vi "运维调试_五参数.vi"(11 "编号":string) -> ()   [LabVIEW 2016, in "斯坦道多参数.lvlib"]
uses:
  <vilib>/Utility/miscctls.llb/LVPointTypeDef.ctl
  <vilib>/Plasmionique/MB Master/MB_Master/MB_Master.lvclass
  <vilib>/Utility/config.llb/NI_LVConfig.lvlib
  <vilib>/ptbypt/NI_PtbyPt.lvlib
panel:
  in  "探头设置":bool
  in  "量程设置":bool
  out "簇":T1
  in  "传感器系列号":bool
  in  "水样保存组数":dbl caption="水样保存组数:"
  in  "水样稳定时间":dbl caption="水样稳定时间:"
  out "模块版本号":string
  out "权限等级":string
  in  "打开modbus":bool
  out "选项卡控件":enum32{"选项卡 1", "选项卡 2"}(tab)
  in  "VISA资源名称":refnum<visa-resource-name> caption="串口"
  in  "IP":string="localhost" caption="IP:"
  in  "Port":u16=502 caption="Port:"
  in  "自动断线重连":bool=TRUE
  in  "连接方式":u16(ring) items=["Modbus RTU", "Modbus TCP"]
  in  "密码锁":bool
  in  "设置页返回":bool
  in  "周期设置":bool
  out "当前串口":string
  out "运行状态":enum16{"空闲", "水样测试", "标样核查"}(ring)
  in  "停止":bool
  in  "标样核查":bool
  in  "水样测试":bool
  in  "设置":bool
  in  "探头校正返回":bool
  in  "探头校正":bool
  # "请设置仪器连接方式"
  # "组"
  # "min"
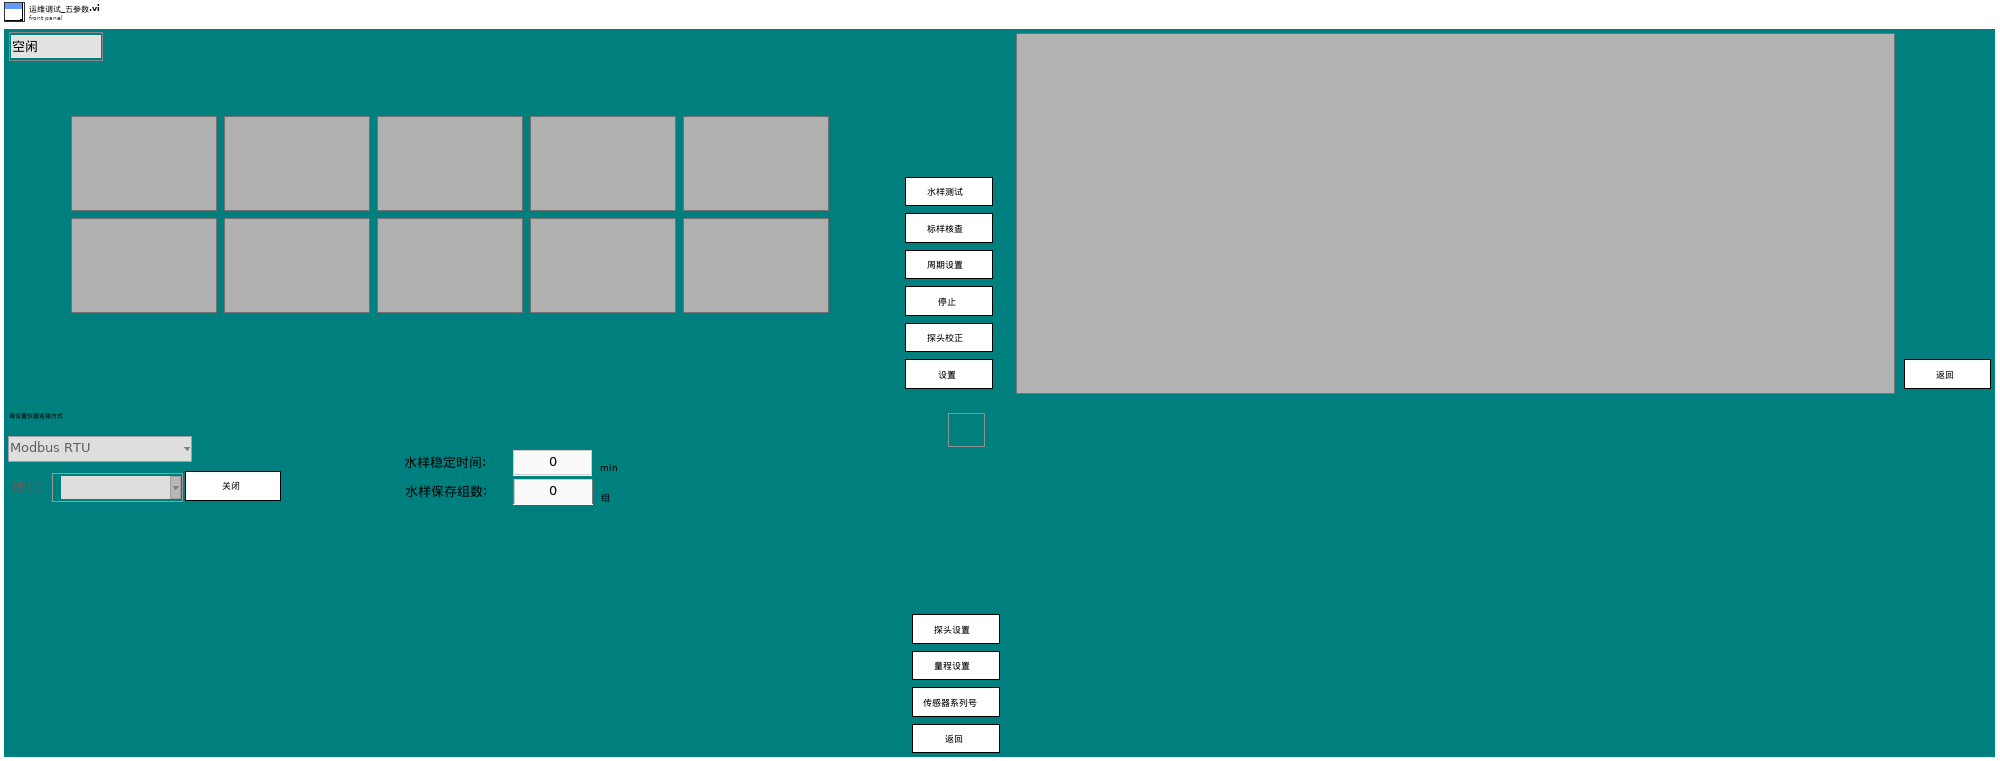
[diagram p1: front panel]
types:
  T1 = typedef "多状态显示框.ctl" = cluster{"多参数状态显示":cluster{"标签":string, "检测值1":cluster{"检测值":dbl, "单位":string, "启用":bool}, "检测值2":cluster{"检测值":dbl, "单位":string, "启用":bool}, "数据标识":string}, "多参数状态显示 2":cluster{"标签":string, "检测值1":cluster{"检测值":dbl, "单位":string, "启用":bool}, "检测值2":cluster{"检测值":dbl, "单位":string, "启用":bool}, "数据标识":string}, "多参数状态显示 3":cluster{"标签":string, "检测值1":cluster{"检测值":dbl, "单位":string, "启用":bool}, "检测值2":cluster{"检测值":dbl, "单位":string, "启用":bool}, "数据标识":string}, "多参数状态显示 4":cluster{"标签":string, "检测值1":cluster{"检测值":dbl, "单位":string, "启用":bool}, "检测值2":cluster{"检测值":dbl, "单位":string, "启用":bool}, "数据标识":string}, "多参数状态显示 5":cluster{"标签":string, "检测值1":cluster{"检测值":dbl, "单位":string, "启用":bool}, "检测值2":cluster{"检测值":dbl, "单位":string, "启用":bool}, "数据标识":string}, "多参数状态显示 6":cluster{"标签":string, "检测值1":cluster{"检测值":dbl, "单位":string, "启用":bool}, "检测值2":cluster{"检测值":dbl, "单位":string, "启用":bool}, "数据标识":string}, "多参数状态显示 7":cluster{"标签":string, "检测值1":cluster{"检测值":dbl, "单位":string, "启用":bool}, "检测值2":cluster{"检测值":dbl, "单位":string, "启用":bool}, "数据标识":string}, "多参数状态显示 8":cluster{"标签":string, "检测值1":cluster{"检测值":dbl, "单位":string, "启用":bool}, "检测值2":cluster{"检测值":dbl, "单位":string, "启用":bool}, "数据标识":string}, "多参数状态显示 9":cluster{"标签":string, "检测值1":cluster{"检测值":dbl, "单位":string, "启用":bool}, "检测值2":cluster{"检测值":dbl, "单位":string, "启用":bool}, "数据标识":string}, "多参数状态显示 10":cluster{"标签":string, "检测值1":cluster{"检测值":dbl, "单位":string, "启用":bool}, "检测值2":cluster{"检测值":dbl, "单位":string, "启用":bool}, "数据标识":string}}
  T2 = typedef "斯坦道多参数.lvlib/数据流类型.ctl" = cluster{"cmd":enum16{"水样测试", "标样核查", "校准状态同步", "停止"}, "data":variant}
  T3 = typedef "LVPointTypeDef.ctl" = cluster{"Horizontal":i16, "Vertical":i16}
  T4 = enum8{"Enabled", "Disabled", "Disabled and Grayed Out"}
  T5 = cluster{"标签":string, "检测值1":cluster{"检测值":dbl, "单位":string, "启用":bool}, "检测值2":cluster{"检测值":dbl, "单位":string, "启用":bool}, "数据标识":string}[]
  T6 = cluster{"标签":string, "检测值1":cluster{"检测值":dbl, "单位":string, "启用":bool}, "检测值2":cluster{"检测值":dbl, "单位":string, "启用":bool}, "数据标识":string}
  T7 = cluster{"CH":u16, "监测值":dbl, "信号值":sgl, "数据标识":string}
  T8 = cluster{"温度测量值":sgl, "测量值":sgl, "温度偏移修正值":sgl, "信号值":sgl, "数据标识":string}
  T9 = cluster{"温度测量值":sgl, "DO%":sgl, "DOmg/L":sgl, "温度偏移修正值":sgl, "数据标识mg/L":string, "数据标识%":string}
  T10 = cluster{"数组[0]":cluster{"标签":string, "检测值1":cluster{"检测值":dbl, "单位":string, "启用":bool}, "检测值2":cluster{"检测值":dbl, "单位":string, "启用":bool}, "数据标识":string}, "数组[1]":cluster{"标签":string, "检测值1":cluster{"检测值":dbl, "单位":string, "启用":bool}, "检测值2":cluster{"检测值":dbl, "单位":string, "启用":bool}, "数据标识":string}, "数组[2]":cluster{"标签":string, "检测值1":cluster{"检测值":dbl, "单位":string, "启用":bool}, "检测值2":cluster{"检测值":dbl, "单位":string, "启用":bool}, "数据标识":string}, "数组[3]":cluster{"标签":string, "检测值1":cluster{"检测值":dbl, "单位":string, "启用":bool}, "检测值2":cluster{"检测值":dbl, "单位":string, "启用":bool}, "数据标识":string}, "数组[4]":cluster{"标签":string, "检测值1":cluster{"检测值":dbl, "单位":string, "启用":bool}, "检测值2":cluster{"检测值":dbl, "单位":string, "启用":bool}, "数据标识":string}, "数组[5]":cluster{"标签":string, "检测值1":cluster{"检测值":dbl, "单位":string, "启用":bool}, "检测值2":cluster{"检测值":dbl, "单位":string, "启用":bool}, "数据标识":string}, "数组[6]":cluster{"标签":string, "检测值1":cluster{"检测值":dbl, "单位":string, "启用":bool}, "检测值2":cluster{"检测值":dbl, "单位":string, "启用":bool}, "数据标识":string}, "数组[7]":cluster{"标签":string, "检测值1":cluster{"检测值":dbl, "单位":string, "启用":bool}, "检测值2":cluster{"检测值":dbl, "单位":string, "启用":bool}, "数据标识":string}, "数组[8]":cluster{"标签":string, "检测值1":cluster{"检测值":dbl, "单位":string, "启用":bool}, "检测值2":cluster{"检测值":dbl, "单位":string, "启用":bool}, "数据标识":string}, "数组[9]":cluster{"标签":string, "检测值1":cluster{"检测值":dbl, "单位":string, "启用":bool}, "检测值2":cluster{"检测值":dbl, "单位":string, "启用":bool}, "数据标识":string}}
  T11 = cluster{"周期设置类型":enum16{"定点启动", "间隔启动"}, "定时功能启用":bool, "定时间隔":u32, "24H周期设置":bool[]}
  T12 = typedef "LVDateTimeRec.ctl" = cluster{"秒数的小数部分":dbl, "秒":i32, "分":i32, "时":i32, "日":i32, "月":i32, "年":i32, "天数（周）":i32, "天数（年）":i32, "DST":i32}
  T13 = cluster{"运行模式":enum16{"维护模式", "常规模式", "应急模式", "质控模式"}, "24H周期设置":bool[]}
  T14 = cluster{"Major":u16, "Minor":u16, "Fix":u16, "Build":u16}
  T15 = typedef "NI_LVConfig.lvlib/Config Data RefNum.ctl" = refnum<k1>
  T16 = enum32{"Bad", "Idle", "Run top level", "Running"}
  T17 = cluster{"ph":bool, "DO":bool, "Cond":bool, "Turb":bool, "叶绿素a":bool, "藻密度":bool, "ORP":bool, "cod":bool, "DO2":bool}
  T18 = cluster{"baud rate (bps)":u32, "stop bits":u16, "parity":u16, "flow control":u16, "timeout":u32, "retries":i32}
  T19 = cluster{"水温 (℃)":cluster{"量程下限":dbl, "量程上限":dbl}, "DO (mg/L)":cluster{"量程下限":dbl, "量程上限":dbl}, "DO (%)":cluster{"量程下限":dbl, "量程上限":dbl}, "pH":cluster{"量程下限":dbl, "量程上限":dbl}, "电导率 (μS/cm)":cluster{"量程下限":dbl, "量程上限":dbl}, "盐度":cluster{"量程下限":dbl, "量程上限":dbl}, "浊度 (NTU)":cluster{"量程下限":dbl, "量程上限":dbl}, "叶绿素a (μg/L)":cluster{"量程下限":dbl, "量程上限":dbl}, "藻密度 (cells/mL)":cluster{"量程下限":dbl, "量程上限":dbl}, "ORP (mV)":cluster{"量程下限":dbl, "量程上限":dbl}}
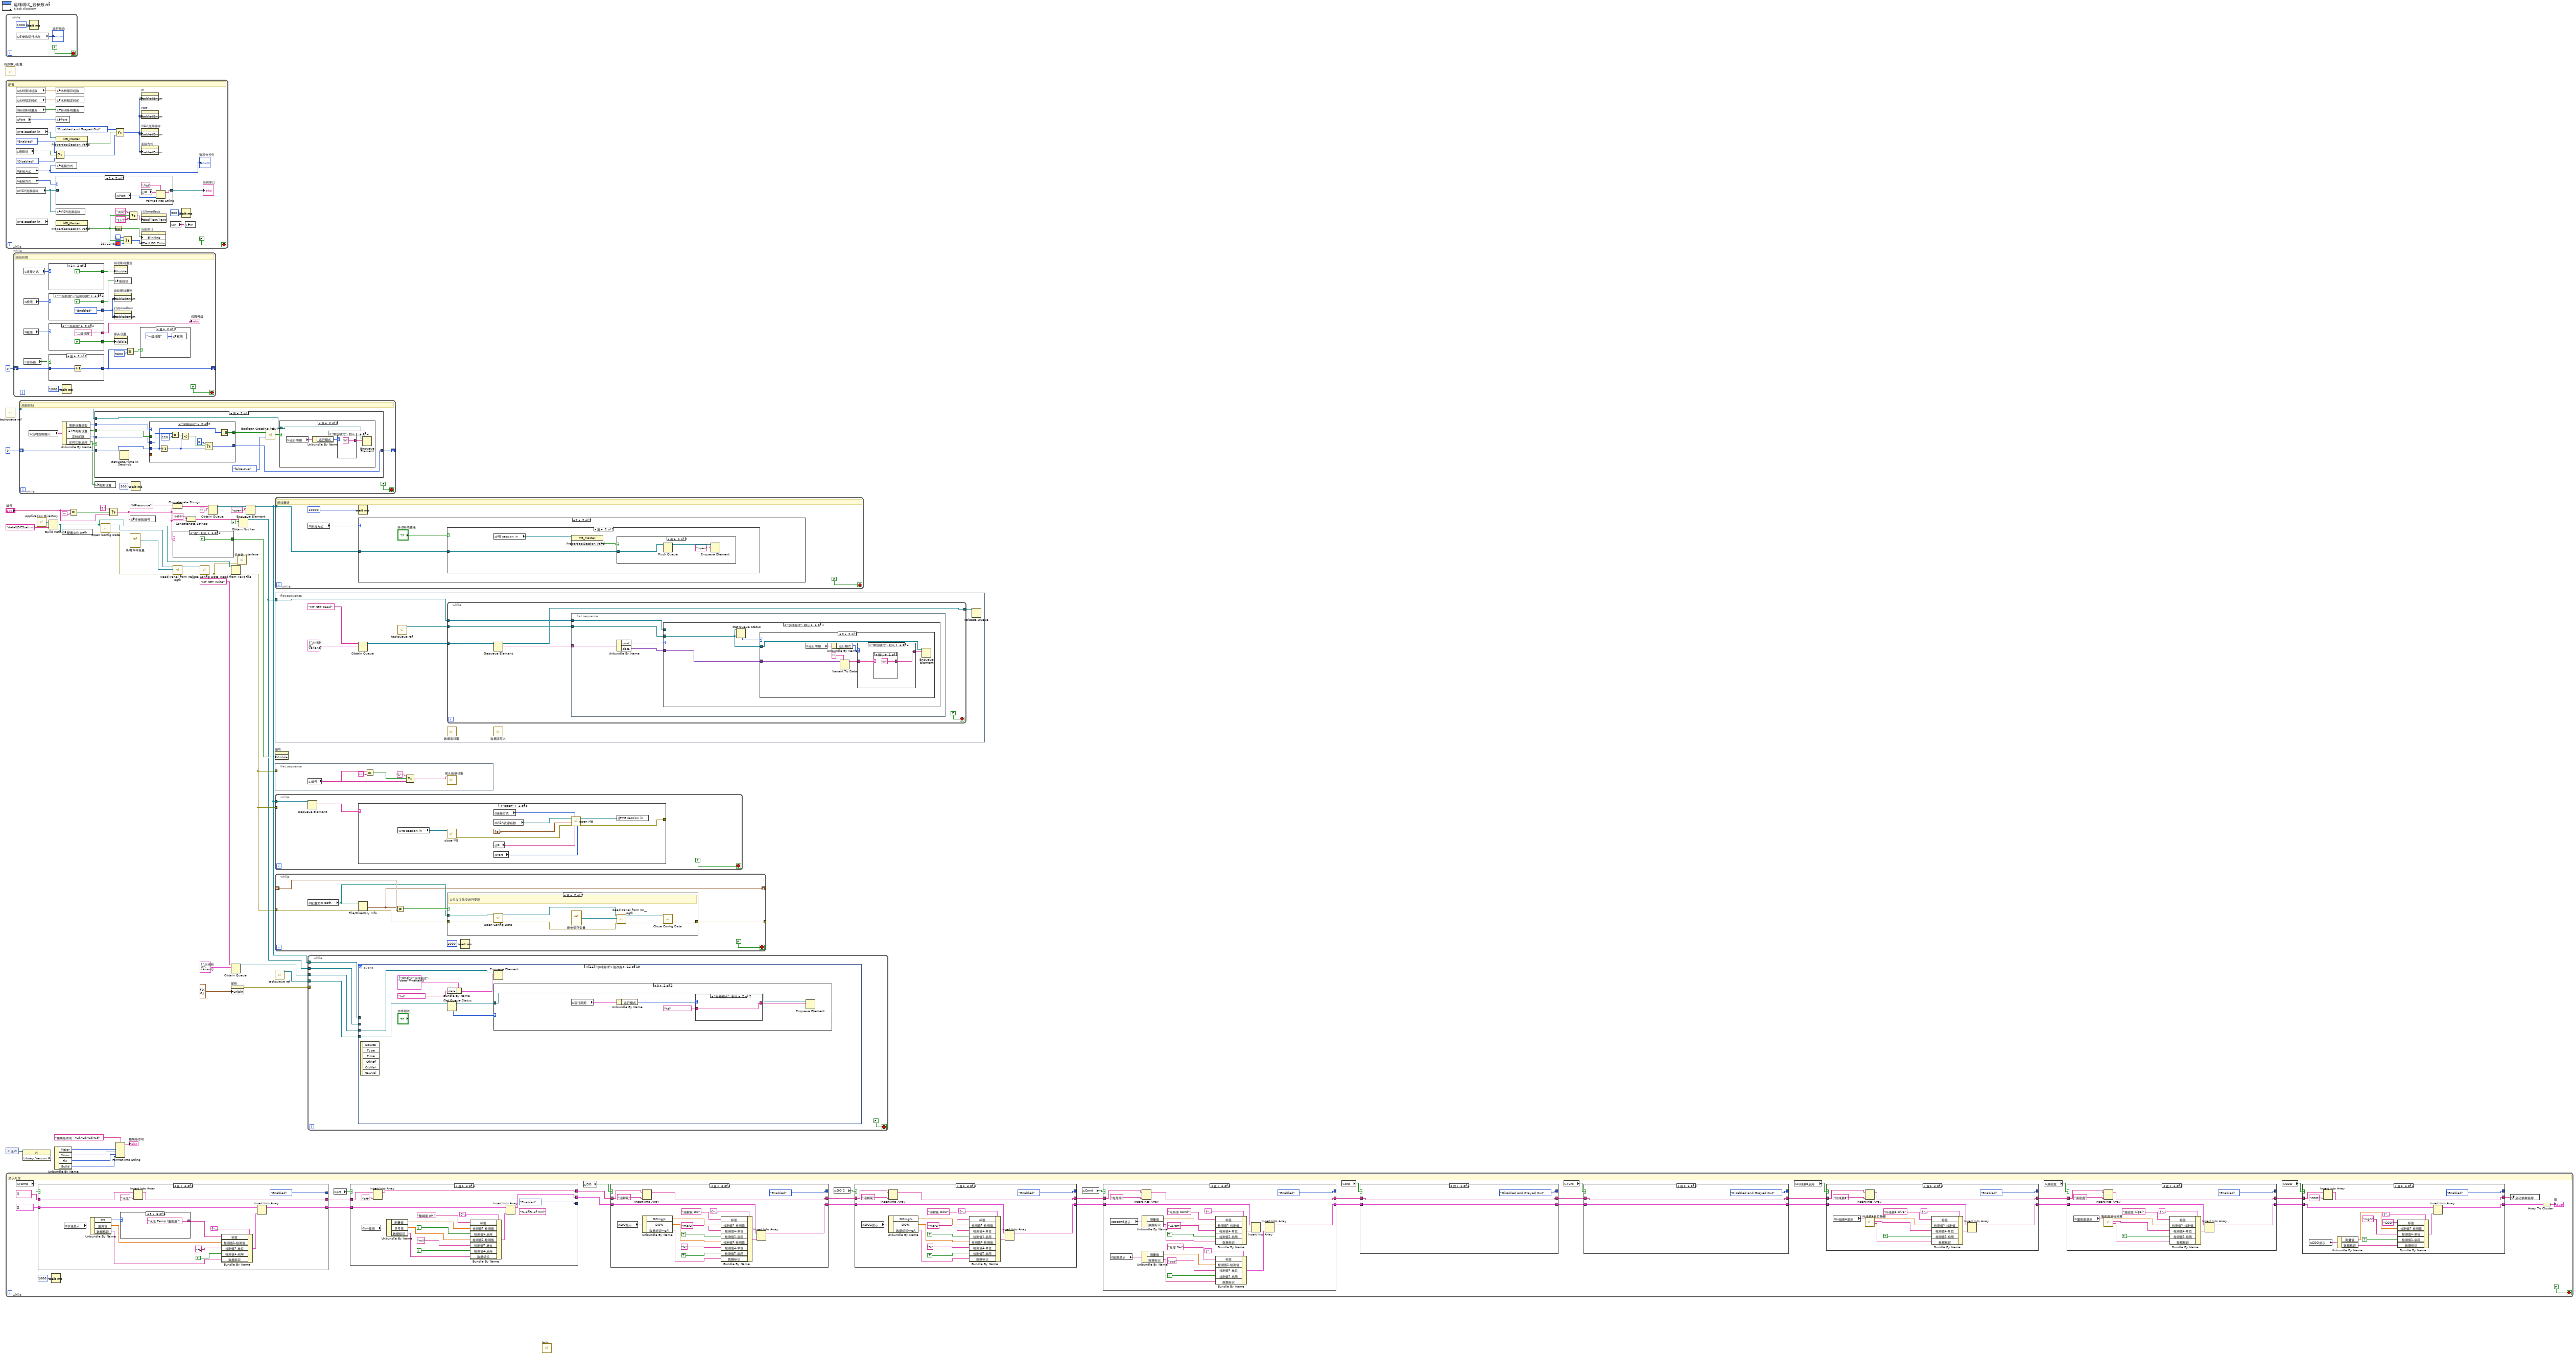
[diagram p0: block diagram]
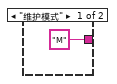
[diagram p3: hidden frame]
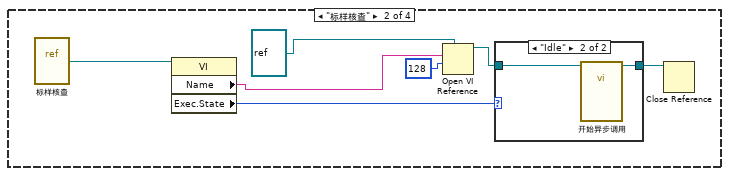
[diagram p5: hidden frame]
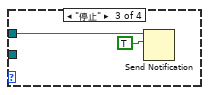
[diagram p7: hidden frame]
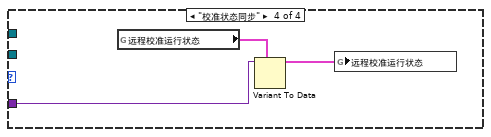
[diagram p8: hidden frame]
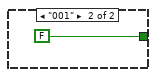
[diagram p9: hidden frame]
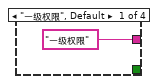
[diagram p17: hidden frame]
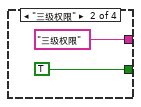
[diagram p18: hidden frame]
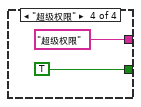
[diagram p19: hidden frame]
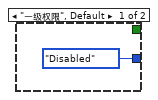
[diagram p20: hidden frame]
diagram:
  n1 = while {
    stop <- FALSE stop-if-true
    n2 = global read "多参数全局变量.vi" "多参数运行状态"() -> (→"运行状态":u16)
    n3 = Wait (ms)(milliseconds to wait=u32 1000 ("等待时间（毫秒）")) -> ()  [unwired: 1 out]
  }
  n4 = call "程序默认配置.vi"() -> ()  [unwired: 11 in, 1 out]
  n5 = while {
    stop <- FALSE stop-if-true
    # "配置"
    n6 = global read "断电保存变量.vi" "水样测试组数"() -> (w47:dbl)
    n7 = global read "断电保存变量.vi" "水样稳定时间"() -> (w49:dbl)
    n8 = global read "断电保存变量.vi" "自动断线重连"() -> (w50:bool)
    n9 = global read "断电保存变量.vi" "Port"() -> (w61:u16)
    n10 = global read "多参数全局变量.vi" "MB session in"() -> (w73:refnum<class "MB_Master.lvclass">)
    n11 = local read "密码锁"() -> (w66:bool)
    n12 = global read "断电保存变量.vi" "连接方式"() -> (w55:u16)
    "选项卡控件" <- w55
    n13 = global read "断电保存变量.vi" "连接方式"() -> (w59:u16)
    n14 = global read "断电保存变量.vi" "VISA资源名称"() -> (w58:refnum<visa-resource-name>)
    n15 = global read "多参数全局变量.vi" "MB session in"() -> (w70:refnum<class "MB_Master.lvclass">)
    n16 = Select(t=T4."Enabled" ("f"), s=w66, f=T4."Disabled") -> (s? t:f=w64:T4)
    n17 = local write "水样保存组数"(w47) -> ()
    n18 = local write "水样稳定时间"(w49) -> ()
    n19 = local write "自动断线重连"(w50) -> ()
    n20 = local write "Port"(w61) -> ()
    n21 = property class="MB_Master"(reference=w73) -> ("Properties:Session Valid"=w72:bool)  [unwired: 1 in, 2 out]
    n22 = local write "连接方式"(w55) -> ()
    n23 = case shown="1" w59 {
      tunnel: w58 -> [w75 _]
      tunnel: [w75 w76] -> w57
      frame 0, Default {
      }
      frame 1 {
        n24 = global read "断电保存变量.vi" "Port"() -> (w77:u16)
        n25 = global read "断电保存变量.vi" "IP"() -> (w79:string)
        n26 = Format Into String(format string=":%d" ("格式字符串"), initial string=w79, w77) -> (resulting string=w76:string)  [unwired: 1 in, 1 out]
      }
    }
    "当前串口" <- w57
    n27 = local write "VISA资源名称"(w58) -> ()
    n28 = property class="MB_Master"(reference=w70) -> ("Properties:Session Valid"=w54:bool)  [unwired: 1 in, 2 out]
    n29 = Not(x=w54) -> (.not. x?=w56:bool)
    n30 = Select(t=T4."Disabled and Grayed Out" ("禁用"), s=w72, f=w64) -> (s? t:f=w60:T4)
    n31 = Select(t=u32 16777216, s=w54, f=u32 16722483) -> (s? t:f=w51:u32)
    n32 = Select(t="关闭" ("布尔文本.文本"), s=w54, f="打开" ("布尔文本.文本")) -> (s? t:f=w67:string)
    n33 = property on="IP" class="Str"("DisabledEnum"=w60) -> ()  [unwired: 2 in, 2 out]
    n34 = property on="Port" class="DigNum (严格)"("DisabledEnum"=w60) -> ()  [unwired: 2 in, 2 out]
    n35 = property on="VISA资源名称" class="VISAName"("DisabledEnum"=w60) -> ()  [unwired: 2 in, 2 out]
    n36 = property on="连接方式" class="Ring (严格)"("DisabledEnum"=w60) -> ()  [unwired: 2 in, 2 out]
    n37 = property on="打开modbus" class="Bool"("BoolText.Text"=w67) -> ()  [unwired: 2 in, 2 out]
    n38 = property on="当前串口" class="Str"("Blinking"=w56, "Text.BG Color"=w51) -> ()  [unwired: 2 in, 2 out]
    n39 = global read "断电保存变量.vi" "IP"() -> (w62:string)
    n40 = Wait (ms)(milliseconds to wait=u32 500 ("等待时间（毫秒）")) -> ()  [unwired: 1 out]
    n41 = local write "IP"(w62) -> ()
  }
  n42 = call "taskqueue ref.vi"() -> ("队列输出"=w4:refnum<queue>)  [unwired: 10 in, 1 out]
  n43 = control-ref of="本VI"() -> (w23:refnum<vi>)
  n44 = while {
    stop <- FALSE stop-if-true
    # "显示处理"
    n45 = global read "断电保存变量.vi" "Temp"() -> (w112:bool)
    n46 = case shown="真" w112 {
      tunnel: [w287 w299] -> w109
      tunnel: T5 [] ("数组") -> [w287 w300]
      tunnel: [T4."Disabled and Grayed Out" ("禁用") T4."Enabled" ("禁用")] -> _
      tunnel: string[] [] -> [w285 w290]
      tunnel: [w285 w289] -> w92
      frame False {
      }
      frame True {
        n47 = global read "多参数全局变量.vi" "水温显示"() -> (w297:T7)
        n48 = Unbundle By Name(w297) -> ("CH"=w296:u16, "监测值"=w294:dbl, "数据标识"=w293:string)
        n49 = case shown="5" w296 {
          tunnel: ["水温 Temp (pH)" ("监测参数1") "水温 Temp (DO)" ("监测参数1") "水温 Temp (浊度)" ("监测参数1") "水温 Temp (电导率)" ("监测参数1") "水温 Temp (叶绿素a)" ("监测参数1") "水温 Temp (藻密度)" ("监测参数1")] -> w302
          frame 0, Default {
          }
          frame 1 {
          }
          frame 2 {
          }
          frame 3 {
          }
          frame 4 {
          }
          frame 5 {
          }
        }
        n50 = Insert Into Array(array=w290, new element="水温" ("新元素/子数组")) -> (w289:string[])  [unwired: 1 in]
        n51 = Bundle By Name(cluster=T6 {"标签"="", "检测值1"={"检测值"=0.0, "单位"="", "启用"=FALSE}, "检测值2"={"检测值"=0.0, "单位"="", "启用"=FALSE}, "数据标识"=""} ("多参数状态显示"), "标签"=w302, "检测值1.检测值"=w294, "检测值1.单位"="℃", "检测值1.启用"=TRUE, "数据标识"=w293) -> (w301:T6)
        n52 = Insert Into Array(array=w300, new element=w301) -> (w299:T5)  [unwired: 1 in]
      }
    }
    n53 = Wait (ms)(milliseconds to wait=u32 1000 ("等待时间（毫秒）")) -> ()  [unwired: 1 out]
    n54 = global read "断电保存变量.vi" "pH"() -> (w110:bool)
    n55 = case shown="真" w110 {
      tunnel: [w268 w283] -> w107
      tunnel: w109 -> [w268 w284]
      tunnel: [T4."Disabled and Grayed Out" ("禁用") T4."Enabled" ("禁用")] -> _
      tunnel: w92 -> [w266 w271]
      tunnel: [w266 w270] -> w91
      frame False {
      }
      frame True {
        (unwired) "%.2f(%.2f mV)" ("格式字符串")
        n56 = global read "多参数全局变量.vi" "ph显示"() -> (w281:T8)
        n57 = Insert Into Array(array=w271, new element="pH" ("新元素/子数组")) -> (w270:string[])  [unwired: 1 in]
        n58 = Unbundle By Name(w281) -> ("测量值"=w278:sgl, "信号值"=w276:sgl, "数据标识"=w274:string)
        n59 = Bundle By Name(cluster=T6 {"标签"="", "检测值1"={"检测值"=0.0, "单位"="", "启用"=FALSE}, "检测值2"={"检测值"=0.0, "单位"="", "启用"=FALSE}, "数据标识"=""} ("多参数状态显示"), "标签"="酸碱度 pH" ("监测参数2"), "检测值1.检测值"=w278, "检测值1.启用"=TRUE, "检测值2.检测值"=w276, "检测值2.单位"="mV", "检测值2.启用"=TRUE, "数据标识"=w274) -> (w272:T6)
        n60 = Insert Into Array(array=w284, new element=w272) -> (w283:T5)  [unwired: 1 in]
      }
    }
    n61 = global read "断电保存变量.vi" "DO"() -> (w108:bool)
    n62 = case shown="真" w108 {
      tunnel: [w248 w264] -> w83
      tunnel: w107 -> [w248 w265]
      tunnel: [T4."Disabled and Grayed Out" ("禁用") T4."Enabled" ("禁用")] -> _
      tunnel: w91 -> [w246 w251]
      tunnel: [w246 w250] -> w82
      frame False {
      }
      frame True {
        n63 = global read "多参数全局变量.vi" "DO显示"() -> (w262:T9)
        n64 = Insert Into Array(array=w251, new element="溶解氧" ("新元素/子数组")) -> (w250:string[])  [unwired: 1 in]
        n65 = Unbundle By Name(w262) -> ("DOmg/L"=w259:sgl, "DO%"=w257:sgl, "数据标识mg/L"=w256:string)
        n66 = Bundle By Name(cluster=T6 {"标签"="", "检测值1"={"检测值"=0.0, "单位"="", "启用"=FALSE}, "检测值2"={"检测值"=0.0, "单位"="", "启用"=FALSE}, "数据标识"=""} ("多参数状态显示"), "标签"="溶解氧 DO" ("监测参数2"), "检测值1.检测值"=w259, "检测值1.单位"="mg/L", "检测值1.启用"=TRUE, "检测值2.检测值"=w257, "检测值2.单位"="%", "检测值2.启用"=TRUE, "数据标识"=w256) -> (w252:T6)
        n67 = Insert Into Array(array=w265, new element=w252) -> (w264:T5)  [unwired: 1 in]
      }
    }
    n68 = global read "断电保存变量.vi" "DO 2"() -> (w84:bool)
    n69 = case shown="真" w84 {
      tunnel: [w117 w133] -> w81
      tunnel: w83 -> [w117 w134]
      tunnel: [T4."Disabled and Grayed Out" ("禁用") T4."Enabled" ("禁用")] -> _
      tunnel: w82 -> [w115 w120]
      tunnel: [w115 w119] -> w80
      frame False {
      }
      frame True {
        n70 = global read "多参数全局变量.vi" "DO2显示"() -> (w131:T9)
        n71 = Insert Into Array(array=w120, new element="溶解氧" ("新元素/子数组")) -> (w119:string[])  [unwired: 1 in]
        n72 = Unbundle By Name(w131) -> ("DOmg/L"=w128:sgl, "DO%"=w126:sgl, "数据标识mg/L"=w125:string)
        n73 = Bundle By Name(cluster=T6 {"标签"="", "检测值1"={"检测值"=0.0, "单位"="", "启用"=FALSE}, "检测值2"={"检测值"=0.0, "单位"="", "启用"=FALSE}, "数据标识"=""} ("多参数状态显示"), "标签"="溶解氧 DO2" ("监测参数2"), "检测值1.检测值"=w128, "检测值1.单位"="mg/L", "检测值1.启用"=TRUE, "检测值2.检测值"=w126, "检测值2.单位"="%", "检测值2.启用"=TRUE, "数据标识"=w125) -> (w121:T6)
        n74 = Insert Into Array(array=w134, new element=w121) -> (w133:T5)  [unwired: 1 in]
      }
    }
    n75 = global read "断电保存变量.vi" "Cond"() -> (w106:bool)
    n76 = case shown="真" w106 {
      tunnel: w81 -> [w222 w245]
      tunnel: [w222 w241] -> w98
      tunnel: [T4."Disabled and Grayed Out" ("禁用") T4."Enabled" ("禁用")] -> _
      tunnel: w80 -> [w220 w225]
      tunnel: [w220 w224] -> w90
      frame False {
      }
      frame True {
        n77 = global read "多参数全局变量.vi" "spcond显示"() -> (w243:T8)
        n78 = global read "多参数全局变量.vi" "盐度显示"() -> (w240:T8)
        n79 = Insert Into Array(array=w225, new element="电导率" ("新元素/子数组")) -> (w224:string[])  [unwired: 1 in]
        n80 = Unbundle By Name(w243) -> ("测量值"=w234:sgl, "数据标识"=w232:string)
        n81 = Unbundle By Name(w240) -> ("测量值"=w229:sgl, "数据标识"=w228:string)
        n82 = Bundle By Name(cluster=T6 {"标签"="", "检测值1"={"检测值"=0.0, "单位"="", "启用"=FALSE}, "检测值2"={"检测值"=0.0, "单位"="", "启用"=FALSE}, "数据标识"=""} ("多参数状态显示"), "标签"="电导率 Cond" ("监测参数2"), "检测值1.检测值"=w234, "检测值1.单位"="μS/cm", "检测值1.启用"=TRUE, "数据标识"=w232) -> (w231:T6)
        n83 = Bundle By Name(cluster=T6 {"标签"="", "检测值1"={"检测值"=0.0, "单位"="", "启用"=FALSE}, "检测值2"={"检测值"=0.0, "单位"="", "启用"=FALSE}, "数据标识"=""} ("多参数状态显示"), "标签"="盐度 Sal" ("监测参数2"), "检测值1.检测值"=w229, "检测值1.单位"="ppt" ("检测值2.单位"), "检测值1.启用"=TRUE, "数据标识"=w228) -> (w226:T6)
        n84 = Insert Into Array(array=w245, new element=w231) -> (w242:T5)  [unwired: 1 in]
        n85 = Insert Into Array(array=w242, new element=w226) -> (w241:T5)  [unwired: 1 in]
      }
    }
    n86 = global read "断电保存变量.vi" "orp"() -> (w100:bool)
    n87 = case shown="假" w100 {
      tunnel: w98 -> [w154 w168]
      tunnel: [w154 w167] -> w99
      tunnel: [T4."Disabled and Grayed Out" ("禁用") T4."Enabled" ("禁用")] -> _
      tunnel: w90 -> [w152 w157]
      tunnel: [w152 w156] -> w89
      frame False {
      }
      frame True {
        n88 = global read "多参数全局变量.vi" "ORP显示"() -> (w165:T8)
        n89 = Insert Into Array(array=w157, new element="ORP" ("新元素/子数组")) -> (w156:string[])  [unwired: 1 in]
        n90 = Unbundle By Name(w165) -> ("测量值"=w160:sgl, "数据标识"=w159:string)
        n91 = Bundle By Name(cluster=T6 {"标签"="", "检测值1"={"检测值"=0.0, "单位"="", "启用"=FALSE}, "检测值2"={"检测值"=0.0, "单位"="", "启用"=FALSE}, "数据标识"=""} ("多参数状态显示"), "标签"="ORP" ("监测参数2"), "检测值1.检测值"=w160, "检测值1.单位"="mV", "检测值1.启用"=TRUE, "数据标识"=w159) -> (w158:T6)
        n92 = Insert Into Array(array=w168, new element=w158) -> (w167:T5)  [unwired: 1 in]
      }
    }
    n93 = global read "断电保存变量.vi" "Turb"() -> (w105:bool)
    n94 = case shown="假" w105 {
      tunnel: w99 -> [w205 w219]
      tunnel: [w205 w218] -> w104
      tunnel: [T4."Disabled and Grayed Out" ("禁用") T4."Enabled" ("禁用")] -> _
      tunnel: w89 -> [w203 w208]
      tunnel: [w203 w207] -> w88
      frame False {
      }
      frame True {
        n95 = global read "多参数全局变量.vi" "浊度显示"() -> (w216:T8)
        n96 = Insert Into Array(array=w208, new element="浊度" ("新元素/子数组")) -> (w207:string[])  [unwired: 1 in]
        n97 = Unbundle By Name(w216) -> ("测量值"=w211:sgl, "数据标识"=w210:string)
        n98 = Bundle By Name(cluster=T6 {"标签"="", "检测值1"={"检测值"=0.0, "单位"="", "启用"=FALSE}, "检测值2"={"检测值"=0.0, "单位"="", "启用"=FALSE}, "数据标识"=""} ("多参数状态显示"), "标签"="浊度 Turb" ("监测参数2"), "检测值1.检测值"=w211, "检测值1.单位"="NTU", "检测值1.启用"=TRUE, "数据标识"=w210) -> (w209:T6)
        n99 = Insert Into Array(array=w219, new element=w209) -> (w218:T5)  [unwired: 1 in]
      }
    }
    n100 = global read "断电保存变量.vi" "叶绿素a启用"() -> (w103:bool)
    n101 = case shown="真" w103 {
      tunnel: w104 -> [w188 w202]
      tunnel: [w188 w201] -> w101
      tunnel: [T4."Disabled and Grayed Out" ("禁用") T4."Enabled" ("禁用")] -> _
      tunnel: w88 -> [w186 w195]
      tunnel: [w186 w194] -> w87
      frame False {
      }
      frame True {
        n102 = global read "多参数全局变量.vi" "叶绿素a显示"() -> (w192:T8)
        n103 = Insert Into Array(array=w195, new element="叶绿素a" ("新元素/子数组")) -> (w194:string[])  [unwired: 1 in]
        n104 = call "叶绿素a单位换算.vi"("叶绿素a显示"=w192) -> ("数据标识"=w189:string, "检测值1.单位"=w191:string, "测量值"=w190:sgl)  [unwired: 8 in]
        n105 = Bundle By Name(cluster=T6 {"标签"="", "检测值1"={"检测值"=0.0, "单位"="", "启用"=FALSE}, "检测值2"={"检测值"=0.0, "单位"="", "启用"=FALSE}, "数据标识"=""} ("多参数状态显示"), "标签"="叶绿素a Chla" ("监测参数2"), "检测值1.检测值"=w190, "检测值1.单位"=w191, "检测值1.启用"=TRUE, "数据标识"=w189) -> (w196:T6)
        n106 = Insert Into Array(array=w202, new element=w196) -> (w201:T5)  [unwired: 1 in]
      }
    }
    n107 = global read "断电保存变量.vi" "藻密度"() -> (w102:bool)
    n108 = case shown="真" w102 {
      tunnel: w101 -> [w171 w185]
      tunnel: [w171 w184] -> w97
      tunnel: [T4."Disabled and Grayed Out" ("禁用") T4."Enabled" ("禁用")] -> _
      tunnel: w87 -> [w169 w178]
      tunnel: [w169 w177] -> w86
      frame False {
      }
      frame True {
        n109 = global read "多参数全局变量.vi" "藻密度显示"() -> (w175:T8)
        n110 = Insert Into Array(array=w178, new element="藻密度" ("新元素/子数组")) -> (w177:string[])  [unwired: 1 in]
        n111 = call "藻密度单位换算.vi"("藻密度显示"=w175) -> ("数据标识"=w173:string, "检测值1.单位"=w172:string, "测量值"=w174:sgl)  [unwired: 8 in]
        n112 = Bundle By Name(cluster=T6 {"标签"="", "检测值1"={"检测值"=0.0, "单位"="", "启用"=FALSE}, "检测值2"={"检测值"=0.0, "单位"="", "启用"=FALSE}, "数据标识"=""} ("多参数状态显示"), "标签"="藻密度 Algal" ("监测参数2"), "检测值1.检测值"=w174, "检测值1.单位"=w172, "检测值1.启用"=TRUE, "数据标识"=w173) -> (w179:T6)
        n113 = Insert Into Array(array=w185, new element=w179) -> (w184:T5)  [unwired: 1 in]
      }
    }
    n114 = global read "断电保存变量.vi" "COD"() -> (w96:bool)
    n115 = case shown="真" w96 {
      tunnel: w97 -> [w137 w151]
      tunnel: [w137 w150] -> w95
      tunnel: [T4."Disabled and Grayed Out" ("禁用") T4."Enabled" ("禁用")] -> _
      tunnel: w86 -> [w135 w140]
      tunnel: [w135 w139] -> w85
      frame False {
      }
      frame True {
        n116 = global read "多参数全局变量.vi" "COD显示"() -> (w148:T8)
        n117 = Insert Into Array(array=w140, new element="COD" ("新元素/子数组")) -> (w139:string[])  [unwired: 1 in]
        n118 = Unbundle By Name(w148) -> ("测量值"=w143:sgl, "数据标识"=w142:string)
        n119 = Bundle By Name(cluster=T6 {"标签"="", "检测值1"={"检测值"=0.0, "单位"="", "启用"=FALSE}, "检测值2"={"检测值"=0.0, "单位"="", "启用"=FALSE}, "数据标识"=""} ("多参数状态显示"), "标签"="COD" ("监测参数2"), "检测值1.检测值"=w143, "检测值1.单位"="mg/L", "检测值1.启用"=TRUE, "数据标识"=w142) -> (w141:T6)
        n120 = Insert Into Array(array=w151, new element=w141) -> (w150:T5)  [unwired: 1 in]
      }
    }
    n121 = global write "多参数全局变量.vi" "启动参数名称"(w85) -> ()
    n122 = Array To Cluster(array=w95) -> (cluster=→"簇":T10)
  }
  n123 = while {
    shift-right: [w319] -> _
    shift-left: u32 0 ("等待时间（毫秒）") -> [w320]
    stop <- FALSE stop-if-true
    # "密码权限"
    n124 = local read "连接方式"() -> (w316:u16)
    n125 = global read "多参数全局变量.vi" "权限"() -> (w311:enum16{"一级权限", "二级权限", "三级权限", "超级权限"})
    n126 = global read "多参数全局变量.vi" "权限"() -> (w312:enum16{"一级权限", "二级权限", "三级权限", "超级权限"})
    n127 = local read "密码锁"() -> (w321:bool)
    n128 = case shown="1" w316 {
      tunnel: [_ TRUE ("可见")] -> w315
      frame 0, Default {
      }
      frame 1 {
      }
    }
    n129 = case shown="\"二级权限\"..\"超级权限\"" w311 {
      tunnel: [T4."Disabled" ("禁用") T4."Enabled" ("禁用")] -> w314
      tunnel: [_ TRUE ("可见")] -> w309
      frame "一级权限", Default {
      }
      frame "二级权限".."超级权限" {
      }
    }
    n130 = case shown="\"二级权限\"" w312 {
      tunnel: ["一级权限" ("权限等级") "三级权限" ("权限等级") "二级权限" ("权限等级") "超级权限" ("权限等级")] -> w313
      tunnel: [_ TRUE FALSE TRUE] -> w310
      frame "一级权限", Default {
      }
      frame "三级权限" {
      }
      frame "二级权限" {
      }
      frame "超级权限" {
      }
    }
    "权限等级" <- w313
    n131 = case shown="真" w321 {
      tunnel: w320 -> [_ w327]
      tunnel: [_ w326] -> w319
      frame False {
      }
      frame True {
        n132 = Increment(x=w327) -> (x+1=w326:u32)
      }
    }
    n133 = Wait (ms)(milliseconds to wait=u32 1000 ("等待时间（毫秒）")) -> ()  [unwired: 1 out]
    n134 = property on="自动断线重连" class="Bool (严格)"("Visible"=w315) -> ()  [unwired: 2 in, 2 out]
    n135 = local write "密码锁"(w309) -> ()
    n136 = property on="自动断线重连" class="Bool (严格)"("DisabledEnum"=w314) -> ()  [unwired: 2 in, 2 out]
    n137 = property on="打开modbus" class="Bool"("DisabledEnum"=w314) -> ()  [unwired: 2 in, 2 out]
    n138 = property on="探头设置" class="Bool"("Visible"=w310) -> ()  [unwired: 2 in, 2 out]
    n139 = Greater Or Equal?(x=w319, y=u32 3600) -> (x >= y?=w317:bool)
    n140 = case shown="真" w317 {
      frame False {
      }
      frame True {
        n141 = global write "多参数全局变量.vi" "权限"(enum16{"一级权限", "二级权限", "三级权限", "超级权限"}."一级权限" ("权限")) -> ()
      }
    }
  }
  n142 = while {
    shift-right: [w340] -> _
    shift-left: u32 0 ("等待时间（毫秒）") -> [w341]
    tunnel: w4 -> [w338]
    stop <- FALSE stop-if-true
    # "周期控制"
    n143 = global read "断电保存变量.vi" "定时控制输入"() -> (w343:T11)
    n144 = Unbundle By Name(w343) -> ("周期设置类型"=w345:enum16{"定点启动", "间隔启动"}, "24H周期设置"=w344:bool[], "定时间隔"=w342:u32, "定时功能启用"=w339:bool)
    n145 = case shown="真" w339 {
      tunnel: w345 -> [_ w356]
      tunnel: w344 -> [_ w355]
      tunnel: w342 -> [_ w354]
      tunnel: w341 -> [_ w353]
      tunnel: [_ w352] -> w340
      tunnel: w338 -> [_ w351]
      frame False {
      }
      frame True {
        n146 = Get Date/Time In Seconds() -> (seconds since 1Jan1904=w357:timestamp)
        n147 = case shown="\"间隔启动\"" w356 {
          tunnel: w357 -> [w373 _]
          tunnel: w355 -> [w370 _]
          tunnel: [w364 w381] -> w350
          tunnel: w354 -> [_ w380]
          tunnel: w353 -> [_ w382]
          tunnel: [_ w376] -> w352
          frame "定点启动", Default {
            n148 = Seconds To Date/Time(time stamp (now)=w373) -> (date time rec=w372:T12)  [unwired: 1 in]
            n149 = Unbundle By Name(w372) -> ("时"=w371:i32, "分"=w369:i32, "秒"=w368:i32)
            n150 = Equal To 0?(x=w369) -> (x = 0?=w366:bool)
            n151 = Equal To 0?(x=w368) -> (x = 0?=w365:bool)
            n152 = Index Array(array=w370, index=w371) -> (element=w367:bool)
            n153 = Compound Arithmetic op=AND ("复合运算")(w367, w366, w365) -> (w364:bool)
          }
          frame "间隔启动" {
            n154 = Increment(x=w382) -> (x+1=w375:u32)
            n155 = Multiply(x=w380, y=u32 120) -> (x*y=w374:u32)
            n156 = Less?(x=w374, y=w375) -> (x < y?=w378:bool)
            n157 = Select(t=u32 0 ("y"), s=w378, f=w375) -> (s? t:f=w376:u32)
            n158 = Equal To 0?(x=w382) -> (x = 0?=w381:bool)
          }
        }
        n159 = call <vilib>:"Boolean Crossing PtByPt.vi"("direction"=enum16{"either", "false-true", "true-false"}."false-true", "input"=w350) -> ("crossing"=w349:bool)  [unwired: 1 in]
        n160 = case shown="真" w349 {
          tunnel: w351 -> [_ w359]
          frame False {
          }
          frame True {
            n161 = global read "断电保存变量.vi" "运行周期"() -> (w360:T13)
            n162 = Unbundle By Name(w360) -> ("运行模式"=w361:enum16{"维护模式", "常规模式", "应急模式", "质控模式"})
            n163 = case shown="\"常规模式\", 默认" w361 {
              tunnel: ["M" ("数据标记表") "N" ("数据标记表")] -> w358
              frame "维护模式" {
              }
              frame "常规模式", Default {
              }
            }
            n164 = Enqueue Element(queue=w359, element=w358) -> ()  [unwired: 2 in, 3 out]
          }
        }
      }
    }
    n165 = local write "周期设置"(w339) -> ()
    n166 = Wait (ms)(milliseconds to wait=u32 500 ("等待时间（毫秒）")) -> ()  [unwired: 1 out]
  }
  n167 = property class="VI"(reference=w23) -> ("Library.Version"=w22:T14)  [unwired: 1 in, 2 out]
  n168 = call <vilib>:"Application Directory.vi"() -> ("Application Directory"=w6:path)
  n169 = Build Path(base path=w6, name or relative path="data\\DCSset.ini" ("名称或相对路径")) -> (appended path=w10:path)
  n170 = Unbundle By Name(w22) -> ("Major"=w20:u16, "Minor"=w19:u16, "Fix"=w18:u16, "Build"=w17:u16)
  n171 = global write "多参数全局变量.vi" "配置文件 path"(w10) -> ()
  n172 = Equal?(x="编号", y="") -> (x = y?=w14:bool)
  n173 = call <vilib>:"Open Config Data.vi"("configuration file path"=w10) -> ("error out"=w29:errorcluster, "refnum"=w30:T15)  [unwired: 8 in, 1 out]
  n174 = Select(t="1", s=w14, f="编号") -> (s? t:f=w12:string)
  n175 = Format Into String(format string="模块版本号：%d.%d.%d.%d" ("格式字符串"), w20, w19, w18, w17) -> (resulting string=→"模块版本号":string)  [unwired: 2 in, 1 out]
  n176 = global write "多参数全局变量.vi" "多参数编号"(w12) -> ()
  n177 = vi-ref "断电保存变量.vi"() -> (w26:refnum<vi>)
  n178 = Concatenate Strings("MPresource" ("名称（未命名）"), w12) -> (w36:string)
  n179 = case shown="\"假\", 默认" w12 {
    tunnel: [TRUE ("可见") FALSE ("可见")] -> w24
    frame "假", Default {
    }
    frame "001" {
    }
  }
  n180 = call <userlib>:"Read Panel from INI__ogtk.vi"("error in (no error)"=w29, "VI ref"=w26, "refnum"=w30) -> ("error out"=w27:errorcluster, "refnum out"=w28:T15)  [unwired: 7 in]
  n181 = Concatenate Strings("MPP" ("名称（未命名）"), w12) -> (w37:string)
  n182 = call <vilib>:"Close Config Data.vi"("error in (no error)"=w27, "refnum"=w28) -> ("error out"=w1:errorcluster)  [unwired: 8 in, 1 out]
  n183 = Obtain Queue(name (unnamed)=w36, element data type="" ("名称（未命名）")) -> (queue out=w33:refnum<queue>)  [unwired: 3 in, 2 out]
  n184 = Read from Text File(file (use dialog)=w10, error in=w1) -> (error out=w2:errorcluster)  [unwired: 2 in, 3 out]
  n185 = Obtain Queue(name (unnamed)="MT NET Write" ("名称（未命名）"), element data type=T2 {"cmd"=enum."水样测试", "data"=variant} ("簇")) -> (queue out=w7:refnum<queue>)  [unwired: 3 in, 2 out]
  n186 = property on="窗格" class="Pane"("Origin"=T3 {"Horizontal"=0, "Vertical"=0} ("原点")) -> (error out=w43:errorcluster)  [unwired: 2 in, 1 out]
  n187 = call "多参数 interface.vi"("error in (no error)"=w1) -> ()  [unwired: 11 in]
  n188 = Obtain Notifier(name (unnamed)=w37, notification data type=FALSE) -> (notifier out=w5:refnum<notifier>)  [unwired: 2 in, 2 out]
  n189 = Enqueue Element(queue=w33, element="open" ("元素")) -> (queue out=w32:refnum<queue>)  [unwired: 2 in, 2 out]
  n190 = while {
    tunnel: w32 -> [w386]
    stop <- FALSE stop-if-true
    # "断线重连"
    n191 = global read "断电保存变量.vi" "连接方式"() -> (w387:u16)
    n192 = Wait (ms)(milliseconds to wait=u32 10000 ("等待时间（毫秒）")) -> ()  [unwired: 1 out]
    n193 = case shown="1" w387 {
      tunnel: w386 -> [_ w390]
      frame 0, Default {
      }
      frame 1 {
        n194 = case shown="真" "自动断线重连" {
          tunnel: w390 -> [_ w393]
          frame False {
          }
          frame True {
            n195 = global read "多参数全局变量.vi" "MB session in"() -> (w392:refnum<class "MB_Master.lvclass">)
            n196 = property class="MB_Master"(reference=w392) -> ("Properties:Session Valid"=w391:bool)  [unwired: 1 in, 2 out]
            n197 = case shown="假" w391 {
              tunnel: w393 -> [w394 _]
              frame False {
                n198 = Flush Queue(queue=w394) -> (queue out=w396:refnum<queue>)  [unwired: 1 in, 2 out]
                n199 = Enqueue Element(queue=w396, element="open" ("元素")) -> ()  [unwired: 2 in, 3 out]
              }
              frame True {
              }
            }
          }
        }
      }
    }
  }
  n200 = flat-sequence {
    tunnel: w5 -> [w398]
    frame #0 {
      n201 = Obtain Queue(name (unnamed)="MT NET Read" ("名称（未命名）"), element data type=T2 {"cmd"=enum."水样测试", "data"=variant} ("簇")) -> (queue out=w400:refnum<queue>)  [unwired: 3 in, 2 out]
      n202 = call "taskqueue ref.vi"() -> ("队列输出"=w397:refnum<queue>)  [unwired: 10 in, 1 out]
      n203 = while {
        tunnel: w400 -> [w407]
        tunnel: [w405] -> w401
        tunnel: w398 -> [w404]
        tunnel: w397 -> [w403]
        stop <- FALSE stop-if-true
        n204 = Dequeue Element(queue=w407) -> (queue out=w405:refnum<queue>, element=w406:T2)  [unwired: 2 in, 2 out]
        n205 = flat-sequence {
          tunnel: w406 -> [w413]
          tunnel: w404 -> [w410]
          tunnel: w403 -> [w409]
          frame #0 {
            n206 = Unbundle By Name(w413) -> ("cmd"=w412:enum16{"水样测试", "标样核查", "校准状态同步", "停止"}, "data"=w411:variant)
            n207 = case shown="\"水样测试\", 默认" w412 {
              tunnel: w411 -> [w416 _ _ w443]
              tunnel: w410 -> [_ _ w439 _]
              tunnel: w409 -> [w415 _ _ _]
              frame "水样测试", Default {
                n208 = Get Queue Status(queue=w415) -> (# elements in queue=w414:i32)  [unwired: 2 in, 7 out]
                n209 = case shown="0" w414 {
                  tunnel: w416 -> [_ w421]
                  tunnel: w415 -> [_ w418]
                  frame Default {
                  }
                  frame 0 {
                    n210 = global read "断电保存变量.vi" "运行周期"() -> (w423:T13)
                    n211 = Unbundle By Name(w423) -> ("运行模式"=w422:enum16{"维护模式", "常规模式", "应急模式", "质控模式"})
                    n212 = Variant To Data(type="", Variant=w421) -> (data=w419:string)  [unwired: 1 in, 1 out]
                    n213 = case shown="\"常规模式\", 默认" w422 {
                      tunnel: ["M" ("数据标记表") w426] -> w417
                      tunnel: w419 -> [_ w425]
                      frame "维护模式" {
                      }
                      frame "常规模式", Default {
                        n214 = case shown="默认" w425 {
                          selector: w425 -> [_ w428]
                          tunnel: ["N" ("数据标记表") w428] -> w426
                          frame Default {
                          }
                          frame "hd" {
                          }
                        }
                      }
                    }
                    n215 = Enqueue Element(queue=w418, element=w417) -> ()  [unwired: 2 in, 3 out]
                  }
                }
              }
              frame "标样核查" {
                n216 = vi-ref "标样核查.vi"() -> (w430:refnum<vi>)
                n217 = property class="VI"(reference=w430) -> ("Name"=w434:string, "Exec.State"=w432:T16)  [unwired: 1 in, 2 out]
                n218 = Open VI Reference(type specifier VI Refnum (for type only)=refnum<vi> refnum, vi path=w434, options=128 ("选项")) -> (vi reference=w435:refnum<vi>)  [unwired: 3 in, 1 out]
                n219 = case shown="\"Idle\"" w432 {
                  tunnel: [w436 w438] -> w431
                  tunnel: w435 -> [w436 w437]
                  frame "Bad", Default {
                  }
                  frame "Idle" {
                    n220 = call-by-ref "开始异步调用"(reference=w437) -> (reference out=w438:refnum<vi>)  [unwired: 13 in, 1 out]
                  }
                }
                n221 = Close Reference(reference=w431) -> ()  [unwired: 1 in, 1 out]
              }
              frame "停止" {
                n222 = Send Notification(notification=TRUE ("通知"), notifier=w439) -> ()  [unwired: 1 in, 2 out]
              }
              frame "校准状态同步" {
                n223 = global read "多参数全局变量.vi" "远程校准运行状态"() -> (w442:T17)
                n224 = Variant To Data(type=w442, Variant=w443) -> (data=w441:T17)  [unwired: 1 in, 1 out]
                n225 = global write "多参数全局变量.vi" "远程校准运行状态"(w441) -> ()
              }
            }
          }
        }
      }
      n226 = call "数据流读取.vi"() -> ()  [unwired: 12 in]
      n227 = call "数据流写入.vi"() -> ()  [unwired: 12 in]
      n228 = Release Queue(queue=w401) -> ()  [unwired: 2 in, 3 out]
    }
  }
  n229 = property on="编号" class="Str"("Visible"=w24) -> ()  [unwired: 2 in, 2 out]
  n230 = flat-sequence {
    tunnel: w2 -> [_]
    frame #0 {
      n231 = local read "编号"() -> (w445:string)
      n232 = Equal?(x=w445, y="") -> (x = y?=w447:bool)
      n233 = Select(t="1", s=w447, f=w445) -> (s? t:f=w444:string)
      n234 = call "探头数据读取.vi"("编号"=w444) -> ()  [unwired: 11 in]
    }
  }
  n235 = while {
    tunnel: w32 -> [w450]
    tunnel: w2 -> [_]
    stop <- FALSE stop-if-true
    n236 = Dequeue Element(queue=w450) -> (element=w449:string)  [unwired: 2 in, 3 out]
    n237 = case shown="\"open\"" w449 {
      tunnel: [_ w452 w462] -> _
      frame "假", Default {
      }
      frame "open" {
        n238 = global read "多参数全局变量.vi" "MB session in"() -> (w457:refnum<class "MB_Master.lvclass">)
        n239 = call "close MB.vi"("MB session in"=w457) -> ("error out"=w460:errorcluster)  [unwired: 10 in]
        n240 = global read "断电保存变量.vi" "连接方式"() -> (w455:u16)
        n241 = global read "断电保存变量.vi" "VISA资源名称"() -> (w459:refnum<visa-resource-name>)
        n242 = global read "断电保存变量.vi" "IP"() -> (w454:string)
        n243 = global read "断电保存变量.vi" "Port"() -> (w453:u16)
        n244 = call "open MB.vi"("Port (502)"=w453, "IP Address"=w454, "MODE"=w455, "error in (no error)"=w460, "Serial Config"=T18 {"baud rate (bps)"=9600, "stop bits"=10, "parity"=0, "flow control"=0, "timeout"=1000, "retries"=1}, "VISA资源名称"=w459) -> ("error out"=w452:errorcluster, "MB session out"=w456:refnum<class "MB_Master.lvclass">)  [unwired: 4 in]
        n245 = global write "多参数全局变量.vi" "MB session in"(w456) -> ()
      }
      frame "close" {
        n246 = global read "多参数全局变量.vi" "MB session in"() -> (w461:refnum<class "MB_Master.lvclass">)
        n247 = call "close MB.vi"("MB session in"=w461) -> ("error out"=w462:errorcluster)  [unwired: 10 in]
      }
    }
  }
  n248 = while {
    tunnel: [w470] -> _
    shift-right: [w463] -> _
    shift-left: _ -> [w468]
    tunnel: w2 -> [w465]
    stop <- FALSE stop-if-true
    n249 = global read "多参数全局变量.vi" "配置文件 path"() -> (w464:path)
    n250 = File/Directory Info(path=w464, error in=w465) -> (last mod=w463:timestamp, error out=w466:errorcluster)  [unwired: 5 out]
    n251 = Not Equal?(x=w463, y=w468) -> (x != y?=w467:bool)
    n252 = case shown="真" w467 {
      tunnel: [w472 w480] -> w470
      tunnel: w466 -> [w472 w479]
      tunnel: w464 -> [_ w473]
      frame False {
      }
      frame True {
        # "文件发生改变进行更新"
        n253 = call <vilib>:"Open Config Data.vi"("error in (no error)"=w479, "configuration file path"=w473) -> ("error out"=w478:errorcluster, "refnum"=w477:T15)  [unwired: 7 in, 1 out]
        n254 = vi-ref "断电保存变量.vi"() -> (w474:refnum<vi>)
        n255 = call <userlib>:"Read Panel from INI__ogtk.vi"("error in (no error)"=w478, "VI ref"=w474, "refnum"=w477) -> ("error out"=w476:errorcluster, "refnum out"=w475:T15)  [unwired: 7 in]
        n256 = call <vilib>:"Close Config Data.vi"("error in (no error)"=w476, "refnum"=w475) -> ("error out"=w480:errorcluster)  [unwired: 8 in, 1 out]
      }
    }
    n257 = Wait (ms)(milliseconds to wait=u32 1000 ("等待时间（毫秒）")) -> ()  [unwired: 1 out]
  }
  n258 = call "taskqueue ref.vi"() -> ("队列输出"=w3:refnum<queue>)  [unwired: 10 in, 1 out]
  n259 = while {
    tunnel: w43 -> [_]
    tunnel: w5 -> [w484]
    tunnel: w32 -> [w483]
    tunnel: w7 -> [w482]
    tunnel: w3 -> [w481]
    stop <- FALSE stop-if-true
    n260 = event shown="[11] \"水样测试\": 值改变" {
      selector: _ -> [_ _ _ _ _ _ _ _ _ _ _ _ _ _ _ _ _ _ _]
      dyn-events: _ -> [_ _ _ _ _ _ _ _ _ _ _ _ _ _ _ _ _ _ _]
      timeout: _ -> [_ _ _ _ _ _ _ _ _ _ _ _ _ _ _ _ _ _ _]
      tunnel: w484 -> [_ _ _ _ _ _ _ _ _ _ _ _ _ w554 _ _ _ _ _]
      tunnel: w483 -> [_ _ _ _ _ _ _ _ _ _ _ _ _ _ _ _ w565 _ _]
      tunnel: w482 -> [_ _ _ _ _ _ _ _ _ _ _ w529 w537 w552 _ _ _ _ _]
      tunnel: w481 -> [_ _ _ _ _ _ _ _ _ _ _ w525 _ _ _ _ _ _ _]
      event Timeout {
        n261 = event-data() -> ()  [unwired: 1 in, 3 out]
      }
      event "探头设置": Value Change {
        n262 = event-data() -> ()  [unwired: 1 in, 6 out]
        n263 = call "探头启用设置.vi"() -> ()  [unwired: 12 in]
      }
      event "量程设置": Value Change {
        n264 = event-data() -> ()  [unwired: 1 in, 6 out]
        n265 = global read "断电保存变量.vi" "量程参数"() -> (w488:T19)
        n266 = call "量程参数设置对话框.vi"("量程参数"=w488) -> ("布尔"=w486:bool, "量程参数 2"=w487:T19)  [unwired: 9 in]
        n267 = case shown="真" w486 {
          tunnel: w487 -> [_ w489]
          frame False {
          }
          frame True {
            n268 = flat-sequence {
              tunnel: w489 -> [w490]
              frame #0 {
                n269 = global write "断电保存变量.vi" "量程参数"(w490) -> ()
              }
              frame #1 {
                n270 = call "配置文件保存.vi"() -> ()  [unwired: 12 in]
              }
            }
          }
        }
      }
      event "传感器系列号": Value Change {
        n271 = event-data() -> ()  [unwired: 1 in, 6 out]
        n272 = call "系列号查询.vi"() -> ()  [unwired: 12 in]
      }
      event "水样稳定时间", "水样保存组数": Mouse Down {
        n273 = event-data() -> ("CtlRef"=w491:refnum<vi>)  [unwired: 1 in, 7 out]
        n274 = property class="DigNum (严格)"(reference=w491) -> (reference out=w494:refnum<vi>, "Value"=w493:dbl)  [unwired: 1 in, 1 out]
        n275 = call "数字键盘.vi"("OldNumber"=w493) -> ("NewNumber"=w492:dbl)  [unwired: 1 in]
        n276 = property class="DigNum (严格)"(reference=w494, "Val(Sgnl)"=w492) -> ()  [unwired: 1 in, 2 out]
      }
      event "VISA资源名称", "打开modbus", "连接方式", "自动断线重连": Mouse Down {
        n277 = event-data() -> ()  [unwired: 1 in, 6 out]
        n278 = local read "密码锁"() -> (w495:bool)
        n279 = case shown="假" w495 {
          frame False {
            n280 = One Button Dialog(message="当前操作权限不足,请提升权限!!!" ("消息")) -> ()  [unwired: 1 in, 1 out]
          }
          frame True {
          }
        }
      }
      event "IP": Mouse Down {
        n281 = event-data() -> ("CtlRef"=w498:refnum<vi>)  [unwired: 1 in, 7 out]
        n282 = property on="IP" class="Str"() -> ("DisabledEnum"=w497:T4)  [unwired: 2 in, 2 out]
        n283 = case shown="\"Disabled and Grayed Out\"" w497 {
          tunnel: w498 -> [w502 _ _]
          frame "Enabled" {
            n284 = property class="Str"(reference=w502) -> (reference out=w501:refnum<vi>, "Value"=w500:string)  [unwired: 1 in, 1 out]
            n285 = call "字符键盘.vi"("Old String"=w500) -> ("String"=w499:string)  [unwired: 10 in]
            n286 = property class="Str"(reference=w501, "Val(Sgnl)"=w499) -> ()  [unwired: 1 in, 2 out]
          }
          frame "Disabled and Grayed Out" {
            n287 = One Button Dialog(message="关闭连接后才可设置!" ("消息")) -> ()  [unwired: 1 in, 1 out]
          }
          frame "Disabled", Default {
            n288 = One Button Dialog(message="当前操作权限不足,请提升权限!!!" ("消息")) -> ()  [unwired: 1 in, 1 out]
          }
        }
      }
      event "Port": Mouse Down {
        n289 = event-data() -> ("CtlRef"=w506:refnum<vi>)  [unwired: 1 in, 7 out]
        n290 = property on="Port" class="DigNum (严格)"() -> ("DisabledEnum"=w505:T4)  [unwired: 2 in, 2 out]
        n291 = case shown="\"Enabled\"" w505 {
          tunnel: w506 -> [w510 _ _]
          frame "Enabled" {
            n292 = property class="DigNum (严格)"(reference=w510) -> (reference out=w509:refnum<vi>, "Value"=w508:u16)  [unwired: 1 in, 1 out]
            n293 = call "数字键盘.vi"("OldNumber"=w508) -> ("NewNumber"=w507:dbl)  [unwired: 1 in]
            n294 = property class="DigNum (严格)"(reference=w509, "Val(Sgnl)"=w507) -> ()  [unwired: 1 in, 2 out]
          }
          frame "Disabled and Grayed Out" {
            n295 = One Button Dialog(message="关闭连接后才可设置!" ("消息")) -> ()  [unwired: 1 in, 1 out]
          }
          frame "Disabled", Default {
            n296 = One Button Dialog(message="当前操作权限不足,请提升权限!!!" ("消息")) -> ()  [unwired: 1 in, 1 out]
          }
        }
      }
      event "密码锁": Value Change {
        n297 = event-data() -> ("NewVal"=w513:bool)  [unwired: 1 in, 5 out]
        n298 = case shown="真" w513 {
          frame False {
            n299 = global write "多参数全局变量.vi" "权限"(enum16{"一级权限", "二级权限", "三级权限"}."一级权限" ("权限")) -> ()
          }
          frame True {
            n300 = global read "多参数全局变量.vi" "权限密码"() -> (w516:u32[])
            n301 = global read "多参数全局变量.vi" "权限"() -> (w515:enum16{"一级权限", "二级权限", "三级权限", "超级权限"})
            n302 = call "密码权限设置.vi"("权限输入"=w515, "权限密码"=w516) -> ("权限"=w517:enum16{"一级权限", "二级权限", "三级权限", "超级权限"})  [unwired: 9 in]
            n303 = global write "多参数全局变量.vi" "权限"(w517) -> ()
          }
        }
      }
      event "权限等级": Mouse Down {
        n304 = event-data() -> ()  [unwired: 1 in, 8 out]
        n305 = global read "多参数全局变量.vi" "权限密码"() -> (w520:u32[])
        n306 = global read "多参数全局变量.vi" "权限"() -> (w518:enum16{"一级权限", "二级权限", "三级权限", "超级权限"})
        n307 = call "密码权限设置.vi"("权限输入"=w518, "权限密码"=w520) -> ("权限"=w519:enum16{"一级权限", "二级权限", "三级权限", "超级权限"})  [unwired: 9 in]
        n308 = global write "多参数全局变量.vi" "权限"(w519) -> ()
      }
      event "周期设置": Mouse Down {
        n309 = event-data() -> ()  [unwired: 1 in, 6 out]
        n310 = flat-sequence {
          frame #0 {
            n311 = global read "断电保存变量.vi" "定时控制输入"() -> (w522:T11)
            n312 = call "周期设置.vi"("定时控制输入"=w522) -> ("定时控制输出"=w521:T11)  [unwired: 10 in]
            n313 = global write "断电保存变量.vi" "定时控制输入"(w521) -> ()
          }
          frame #1 {
            n314 = call "配置文件保存.vi"() -> ()  [unwired: 12 in]
          }
        }
      }
      event "水样测试": Value Change {
        n315 = event-data() -> ()  [unwired: 1 in, 6 out]
        n316 = Bundle By Name(cluster=T2 {"cmd"=enum."水样测试", "data"=variant} ("元素"), "data"="hd" ("数据标记表")) -> (w526:T2)
        n317 = Get Queue Status(queue=w525) -> (queue out=w523:refnum<queue>, # elements in queue=w524:i32)  [unwired: 2 in, 6 out]
        n318 = Enqueue Element(queue=w529, element=w526) -> ()  [unwired: 2 in, 3 out]
        n319 = case shown="0" w524 {
          tunnel: w523 -> [_ w531]
          frame Default {
          }
          frame 0 {
            n320 = global read "断电保存变量.vi" "运行周期"() -> (w534:T13)
            n321 = Unbundle By Name(w534) -> ("运行模式"=w533:enum16{"维护模式", "常规模式", "应急模式", "质控模式"})
            n322 = case shown="\"常规模式\", 默认" w533 {
              tunnel: ["M" ("数据标记表") w536] -> w530
              tunnel: "hd" ("数据标记表") -> [_ w536]
              frame "维护模式" {
              }
              frame "常规模式", Default {
              }
            }
            n323 = Enqueue Element(queue=w531, element=w530) -> ()  [unwired: 2 in, 3 out]
          }
        }
      }
      event "标样核查": Value Change {
        n324 = event-data() -> ()  [unwired: 1 in, 6 out]
        n325 = call "标样核查配置.vi"() -> ("确认输出"=w538:bool)  [unwired: 11 in]
        n326 = case shown="真" w538 {
          tunnel: w537 -> [_ w547]
          frame False {
          }
          frame True {
            n327 = vi-ref "标样核查.vi"() -> (w540:refnum<vi>)
            n328 = Enqueue Element(queue=w547, element=T2 {"cmd"=enum."标样核查", "data"=variant} ("元素")) -> ()  [unwired: 2 in, 3 out]
            n329 = property class="VI"(reference=w540) -> ("Name"=w544:string, "Exec.State"=w542:T16)  [unwired: 1 in, 2 out]
            n330 = Open VI Reference(type specifier VI Refnum (for type only)=refnum<vi> refnum, vi path=w544, options=128 ("选项")) -> (vi reference=w545:refnum<vi>)  [unwired: 3 in, 1 out]
            n331 = case shown="\"Idle\"" w542 {
              tunnel: [w548 w550] -> w541
              tunnel: w545 -> [w548 w549]
              frame "Bad", Default {
              }
              frame "Idle" {
                n332 = call-by-ref "开始异步调用"(reference=w549) -> (reference out=w550:refnum<vi>)  [unwired: 13 in, 1 out]
              }
            }
            n333 = Close Reference(reference=w541) -> ()  [unwired: 1 in, 1 out]
          }
        }
      }
      event "停止": Value Change {
        n334 = event-data() -> ()  [unwired: 1 in, 6 out]
        n335 = Send Notification(notification=TRUE ("通知"), notifier=w554) -> ()  [unwired: 1 in, 2 out]
        n336 = Enqueue Element(queue=w552, element=T2 {"cmd"=enum."停止", "data"=variant} ("元素")) -> ()  [unwired: 2 in, 3 out]
      }
      event "设置": Value Change {
        n337 = event-data() -> ()  [unwired: 1 in, 6 out]
        n338 = global write "多参数全局变量.vi" "当前页面"(enum16{"主页面", "参数页面", "校准页面"}."参数页面" ("当前页面")) -> ()
        n339 = property on="窗格" class="Pane"("Origin"=T3 {"Horizontal"=0, "Vertical"=628} ("原点")) -> ()  [unwired: 2 in, 2 out]
      }
      event "VISA资源名称", "连接方式", "IP", "Port", "自动断线重连", "水样稳定时间", "水样保存组数": Value Change {
        n340 = event-data() -> ()  [unwired: 1 in, 6 out]
        n341 = flat-sequence {
          frame #0 {
            n342 = local read "自动断线重连"() -> (w559:bool)
            n343 = global write "断电保存变量.vi" "自动断线重连"(w559) -> ()
            n344 = global write "断电保存变量.vi" "IP"("IP") -> ()
            n345 = global write "断电保存变量.vi" "连接方式"("连接方式") -> ()
            n346 = global write "断电保存变量.vi" "Port"("Port") -> ()
            n347 = global write "断电保存变量.vi" "VISA资源名称"("VISA资源名称") -> ()
            n348 = global write "断电保存变量.vi" "水样稳定时间"("水样稳定时间") -> ()
            n349 = global write "断电保存变量.vi" "水样测试组数"("水样保存组数") -> ()
          }
          frame #1 {
            n350 = call "配置文件保存.vi"() -> ()  [unwired: 12 in]
          }
          frame #2 {
          }
        }
      }
      event "打开modbus": Value Change {
        n351 = event-data() -> ()  [unwired: 1 in, 6 out]
        n352 = global read "多参数全局变量.vi" "MB session in"() -> (w570:refnum<class "MB_Master.lvclass">)
        n353 = Flush Queue(queue=w565) -> (queue out=w564:refnum<queue>)  [unwired: 1 in, 2 out]
        n354 = property class="MB_Master"(reference=w570) -> ("Properties:Session Valid"=w569:bool)  [unwired: 1 in, 2 out]
        n355 = Select(t="close" ("元素"), s=w569, f="open" ("元素")) -> (s? t:f=w566:string)
        n356 = Enqueue Element(queue=w564, element=w566) -> ()  [unwired: 2 in, 3 out]
      }
      event "探头校正返回", "设置页返回": Value Change {
        n357 = event-data() -> ()  [unwired: 1 in, 6 out]
        n358 = property on="窗格" class="Pane"("Origin"=T3 {"Horizontal"=0, "Vertical"=0} ("原点")) -> ()  [unwired: 2 in, 2 out]
        n359 = global write "多参数全局变量.vi" "当前页面"(enum16{"主页面", "参数页面", "校准页面"}."主页面" ("当前页面")) -> ()
      }
      event "探头校正": Value Change {
        n360 = event-data() -> ()  [unwired: 1 in, 6 out]
        n361 = vi-ref "斯坦道多参数.lvlib:校准UI.vi"() -> (w574:refnum<vi>)
        n362 = property on="窗格" class="Pane"("Origin"=T3 {"Horizontal"=1656, "Vertical"=0} ("原点")) -> ()  [unwired: 2 in, 2 out]
        n363 = global write "多参数全局变量.vi" "当前页面"(enum16{"主页面", "参数页面", "校准页面"}."校准页面" ("当前页面")) -> ()
        n364 = property class="VI"(reference=w574) -> (reference out=w576:refnum<vi>, "Exec.State"=w575:T16)  [unwired: 1 in, 1 out]
        n365 = case shown="\"Bad\", 默认" w575 {
          tunnel: [w580 w582] -> w578
          tunnel: w576 -> [w580 w581]
          frame "Bad", Default {
          }
          frame "Idle" {
            n366 = invoke class="VI" method="Run VI"(reference=w581, "Wait until done"=FALSE ("结束前等待"), "Auto Dispose Ref"=FALSE ("自动销毁引用")) -> (reference out=w582:refnum<vi>)  [unwired: 2 in, 4 out]
          }
        }
        n367 = invoke on="探头校准子面板" class="SubPnl" method="Remove VI"() -> (error out=w577:errorcluster)  [unwired: 3 in, 2 out]
        n368 = invoke on="探头校准子面板" class="SubPnl" method="Insert VI"(error in=w577, "VI Ref"=w578) -> ()  [unwired: 2 in, 4 out]
      }
    }
  }
  n369 = call "task.vi"() -> ()  [unwired: 12 in]
